vi "Update Status.vi"(8 "error in (no error)":errorcluster, 11 "CIF_UI in":refnum<class "CIF_UI.lvclass">) -> (0 "error out":errorcluster, 3 "CIF_UI out":refnum<class "CIF_UI.lvclass">)   [LabVIEW 2021, in "CIF_UI.lvclass"]
uses:
  CIF_UI.lvclass
  CIF_UI.lvclass/CIF_UI.ctl
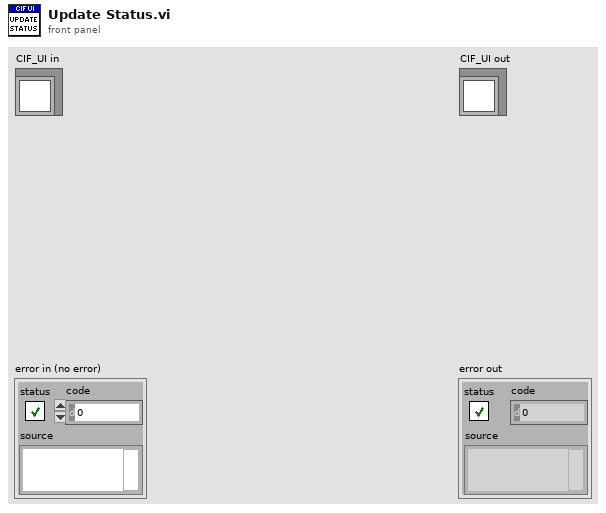
[diagram p1: front panel]
types:
  T1 = typedef "CIF_UI.lvclass/Plugin Summary.ctl" = cluster{"Name":string, "Type":string, "grpc_port":i32, "Version":T2}
  T2 = typedef "CIF_UI.lvclass/Version.ctl" = cluster{"Major":i32, "Minor":i32, "Fix":i32}
  T3 = typedef "CIFCoreChannel_client.lvlib/cif_channelcore_Channel.ctl" = cluster{"name":string, "direction":T4, "type":string, "custom_config":u8[], "connected":bool, "connected_name":string, "forced":bool, "channel_pattern":T5}
  T4 = typedef "CIFCoreChannel_client.lvlib/cif_channelcore_Direction.ctl" = enum32{"PUBLISHER", "SUBSCRIBER"}
  T5 = typedef "CIFCoreChannel_client.lvlib/cif_channelcore_PATTERN.ctl" = enum32{"UNKNOWN", "TAG", "FIFO", "MULTIFIFO", "BACKPRESSUREFIFO"}
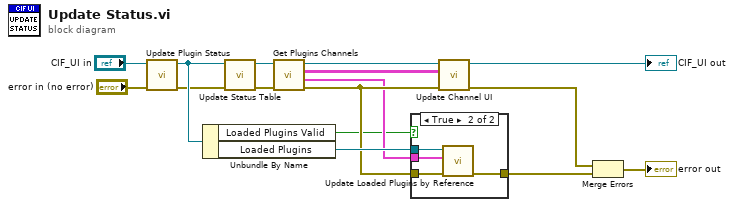
[diagram p0: block diagram]
diagram:
  n1 = call "Update Plugin Status.vi"("error in (no error)"="error in (no error)", "CIF_UI in"="CIF_UI in") -> ("error out"=w6:errorcluster, "CIF_UI out"=w7:refnum<class "CIF_UI.lvclass">)  [unwired: 8 in]
  n2 = Unbundle By Name(w7) -> ("Loaded Plugins Valid"=w3:bool, "Loaded Plugins"=w14:refnum<vi>)
  n3 = call "Update Status Table.vi"("error in (no error)"=w6, "CIFManager_UI in"=w7) -> ("error out"=w5:errorcluster, "CIFManager_UI out"=w4:refnum<class "CIF_UI.lvclass">)  [unwired: 8 in]
  n4 = call "Get Plugins Channels.vi"("error in (no error)"=w5, "CIF_UI in"=w4) -> ("error out"=w13:errorcluster, "Plugin Summary Info"=w8:T1[], "Channels"=w9:T3[][], "CIF_UI out"=w2:refnum<class "CIF_UI.lvclass">)  [unwired: 6 in]
  n5 = case shown="True" w3 {
    tunnel: w14 -> [_ w21]
    tunnel: w13 -> [w17 w20]
    tunnel: [w17 w19] -> w11
    tunnel: w8 -> [_ w18]
    frame False {
    }
    frame True {
      n6 = call "Update Loaded Plugins by Reference.vi"("error in (no error)"=w20, "Plugin Summary Info"=w18, "Loaded Plugins ref in"=w21) -> ("error out"=w19:errorcluster)  [unwired: 7 in, 1 out]
    }
  }
  n7 = call "Update Channel UI.vi"("error in (no error)"=w13, "Channels"=w9, "CIF_UI in"=w2) -> ("error out"=w12:errorcluster, "CIF_UI out"=→"CIF_UI out":refnum<class "CIF_UI.lvclass">)  [unwired: 7 in]
  n8 = Merge Errors(w12, w11) -> (→"error out":errorcluster)
